vi "Read String.vi"(11 "Caraya-TestableClass in":refnum<class "Caraya-TestableClass.lvclass">) -> (2 "String":string, 3 "Caraya-TestableClass out":refnum<class "Caraya-TestableClass.lvclass">)   [LabVIEW 2020, in "Caraya-TestableClass.lvclass"]
uses:
  Caraya-TestableClass.lvclass
  Caraya-TestableClass.lvclass/Caraya-TestableClass.ctl
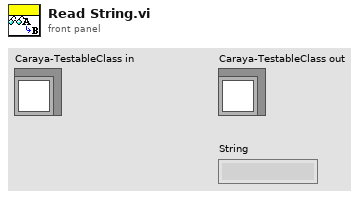
[diagram p1: front panel]
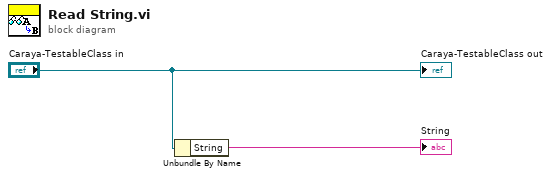
[diagram p0: block diagram]
diagram:
  n1 = Unbundle By Name("Caraya-TestableClass in") -> ("String"=→"String":string)
  "Caraya-TestableClass out" <- "Caraya-TestableClass in"
